vi "Read Counter Driven Output.vi"   [LabVIEW 2017, in "Scan Engine Scripting.lvlib"]
uses:
  Scan Engine Scripting.lvlib
  NI 9475/NI 9475.lvclass
  NI 9474/NI 9474.lvclass
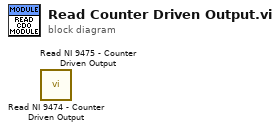
[diagram p0: block diagram]
diagram:
  n1 = call "Read NI 9474 - Counter Driven Output.vi"() -> ()  [unwired: 8 in, 4 out]
  n2 = call "Read NI 9475 - Counter Driven Output.vi"() -> ()  [unwired: 8 in, 4 out]
